vi "数值转换为二进制字符串任意填充.vi"(1 "PadChar":string="0", 2 "Num":u32, 4 "Width":i32=8) -> (6 "BinString":string)   [LabVIEW 2012]
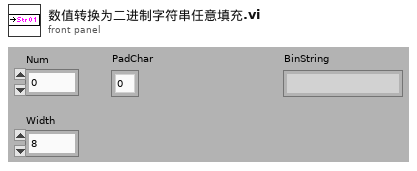
[diagram p1: front panel]
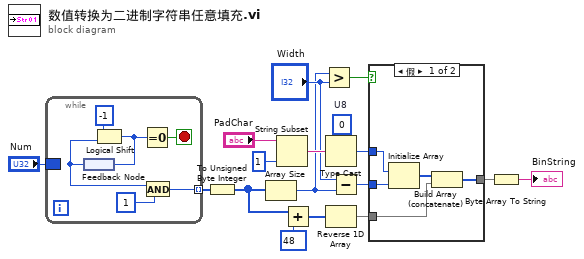
[diagram p0: block diagram]
diagram:
  w11 = u8 0  # U8
  n1 = while {
    tunnel: [w19] -> w15 mode=indexing
    border: "Num" -> [_]
    stop <- w22 stop-if-true
    n2 = feedback #1() -> (w18:u32)
    n3 = Logical Shift(y=i8 -1, x=w18) -> (x << y=w21:u32)
    n4 = feedback-in #1(w21) -> ()
    n5 = Equal To 0?(x=w21) -> (x = 0?=w22:bool)
    n6 = And(x=w18, y=u32 1) -> (x .and. y?=w19:u32)
  }
  n7 = To Unsigned Byte Integer(number=w15) -> (unsigned 8bit integer=w14:u8[])
  n8 = Array Size(array=w14) -> (size(s)=w4:i32)
  n9 = String Subset(string="PadChar", length (rest)=1 ("长度（剩余）")) -> (substring=w12:string)  [unwired: 1 in]
  n10 = Add(x=w14, y=u8 48 ("Width")) -> (x+y=w8:u8[])
  n11 = Greater?(x=w4, y="Width") -> (0:w10:bool)
  n12 = Type Cast(type=w11, x=w12) -> (*(type *) &x=w9:u8)
  n13 = Reverse 1D Array(array=w8) -> (reversed array=w1:u8[])
  n14 = Subtract(x="Width", y=w4) -> (x-y=w3:i32)
  n15 = case shown="假" w10 {
    tunnel: w9 -> [w28 _]
    tunnel: w1 -> [w26 w29]
    tunnel: [w25 w29] -> w7
    tunnel: w3 -> [w24 _]
    frame False {
      n16 = Initialize Array(w28, w24) -> (w27:u8[])
      n17 = Build Array (concatenate)(w27, w26) -> (w25:u8[])
    }
    frame True {
    }
  }
  n18 = Byte Array To String(unsigned byte array=w7) -> (string=→"BinString":string)
